vi "field_sweep_1.vi"() -> ()   [LabVIEW 2016]
uses:
  Controls/State.ctl
  Controls/Data.ctl
  <vilib>/Utility/error.llb/DialogType.ctl
  <vilib>/DAQmx/write.llb/DAQmx Write (Analog DBL 1Chan 1Samp).vi
  <vilib>/DAQmx/create/channels.llb/DAQmx Create Channel (AO-Voltage-Basic).vi
  <vilib>/DAQmx/miscellaneous.llb/DAQmx Fill In Error Info.vi
  <instrlib>/niVNA/niVNA.llb/niVNA Fetch Sweep Measurement (DBL).vi
panel:
  in  "Hysteresis":bool caption="Hysteresis On/Off"
  out "DAQ channel Out":tag="DAQ_6363/ao0"
  in  "Averaging Points":i32=10 min=1 max=3201 step=1
  in  "DAQ channel In":tag="DAQ_6363/ao0"
  in  "Exit Button":bool
  in  "IF Bandwidth":dbl(ring)=1000.0 items=["10 Hz"=10.0, "30 Hz"=30.0, "100 Hz"=100.0, "300 Hz"=300.0, "1 KHz"=1000.0, "3 KHz"=3000.0, "10 KHz"=10000.0, "30 KHz"=30000.0]
  in  "Speed (Oe/sec)":dbl=5.0
  in  "Frequency (Hz)":dbl=3000000000.0 min=10000000.0 max=6000000000.0
  in  "Save Button":bool
  out "Status":string="Shutting down...Sweeping field to zero..."
  out "Cursor":cluster{"x":dbl, "y":dbl} {"x" format="%.2f"; "y" format="%.5f"}
  out "VNA Name Out":refnum<k15>="VNA_5630"
  out "Error Out":errorcluster
  in  "Error In (no error)":errorcluster
  in  "Format":i32(ring)=1 items=["Log Magnitude (dB)"=0, "Lin Magnitude"=1, "Phase (deg)"=2, "VSWR"=3, "Group Delay"=6]
  out "SpectrumGraph":cluster{"Old Field":dbl[], "Old Signal":dbl[]}[](graph)
  in  "S-parameter":i32(ring)=1 caption="Measurement" items=["S11", "S21"]
  in  "Start Button":bool
  in  "Stop Button":bool
  in  "Output Power (dBm)":dbl=1.0 min=-25.0 max=5.0 step=0.5
  in  "Number of Points":i32=1000 min=1 max=3201 step=1
  in  "Stop H Field (Oe)":dbl=1500.0 min=-6000.0 max=6000.0 format="%#_6f"
  in  "Start H Field (Oe)":dbl=1000.0 min=-6000.0 max=6000.0 format="%#_6f"
  in  "VNA Name In":refnum<k15>="VNA_5630"
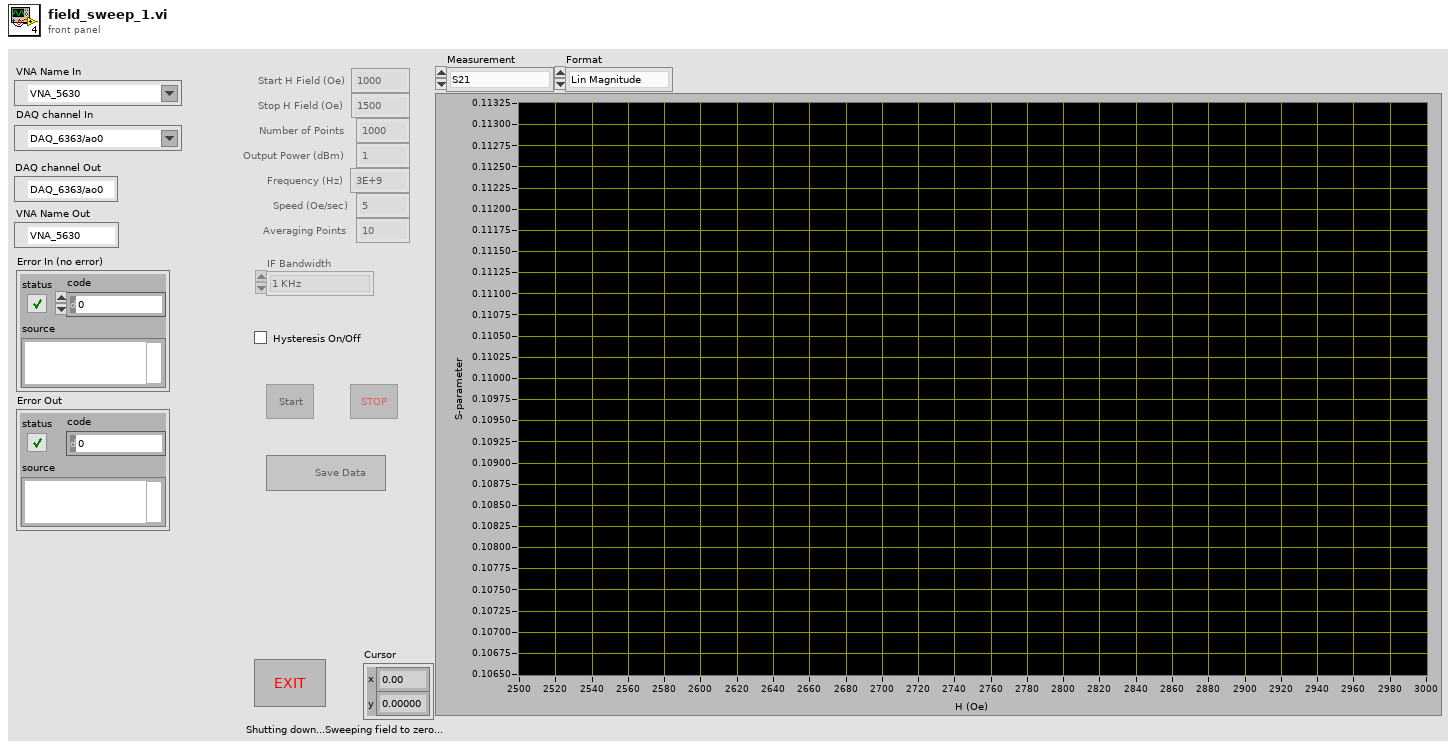
[diagram p1: front panel]
types:
  T1 = typedef "Data.ctl" = cluster{"Field":dbl[], "Signal":dbl[], "Old Field":dbl[], "Old Signal":dbl[]}
  T2 = typedef "State.ctl" = enum16{"Init", "Idle", "Sweeping up", "Sweeping down", "Running", "Shutdown"}
  T3 = typedef "DialogType.ctl" = u16
  T4 = typedef "LVPoint32TypeDef.ctl" = cluster{"Horizontal":i32, "Vertical":i32}
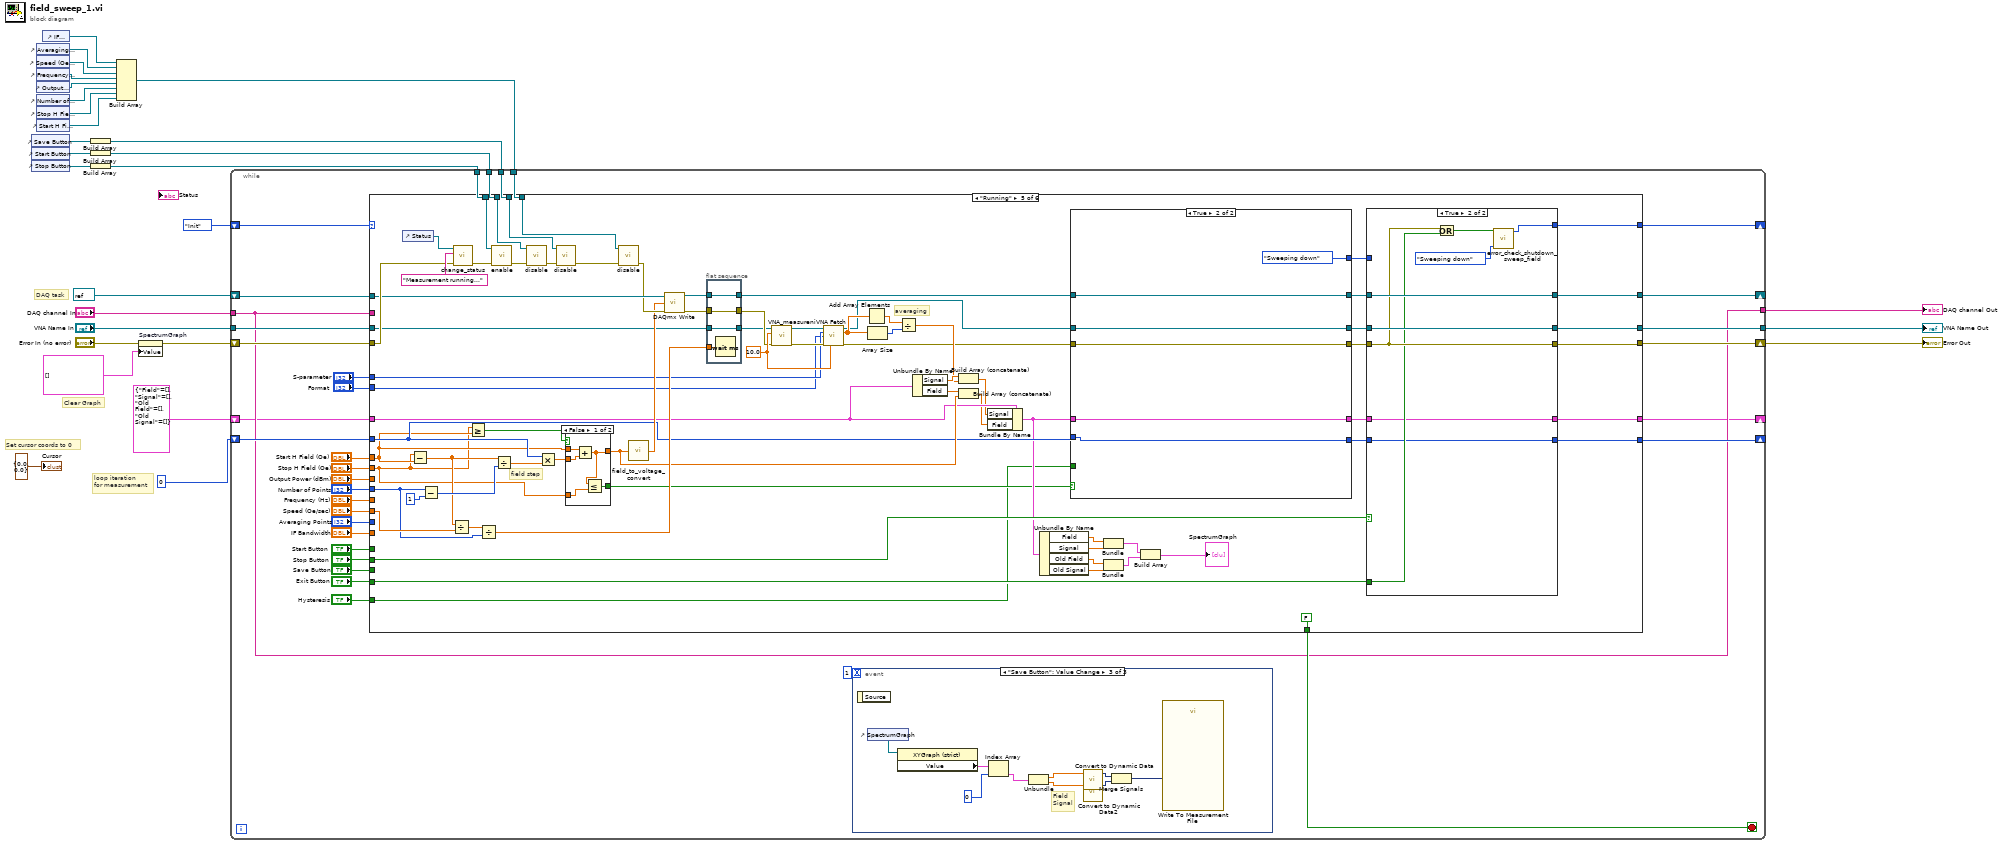
[diagram p0: block diagram]
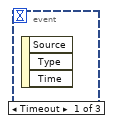
[diagram p2: hidden frame]
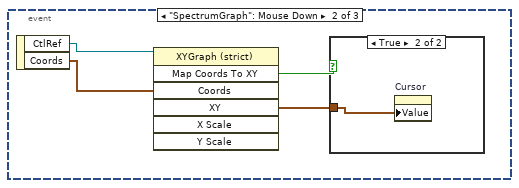
[diagram p3: hidden frame]
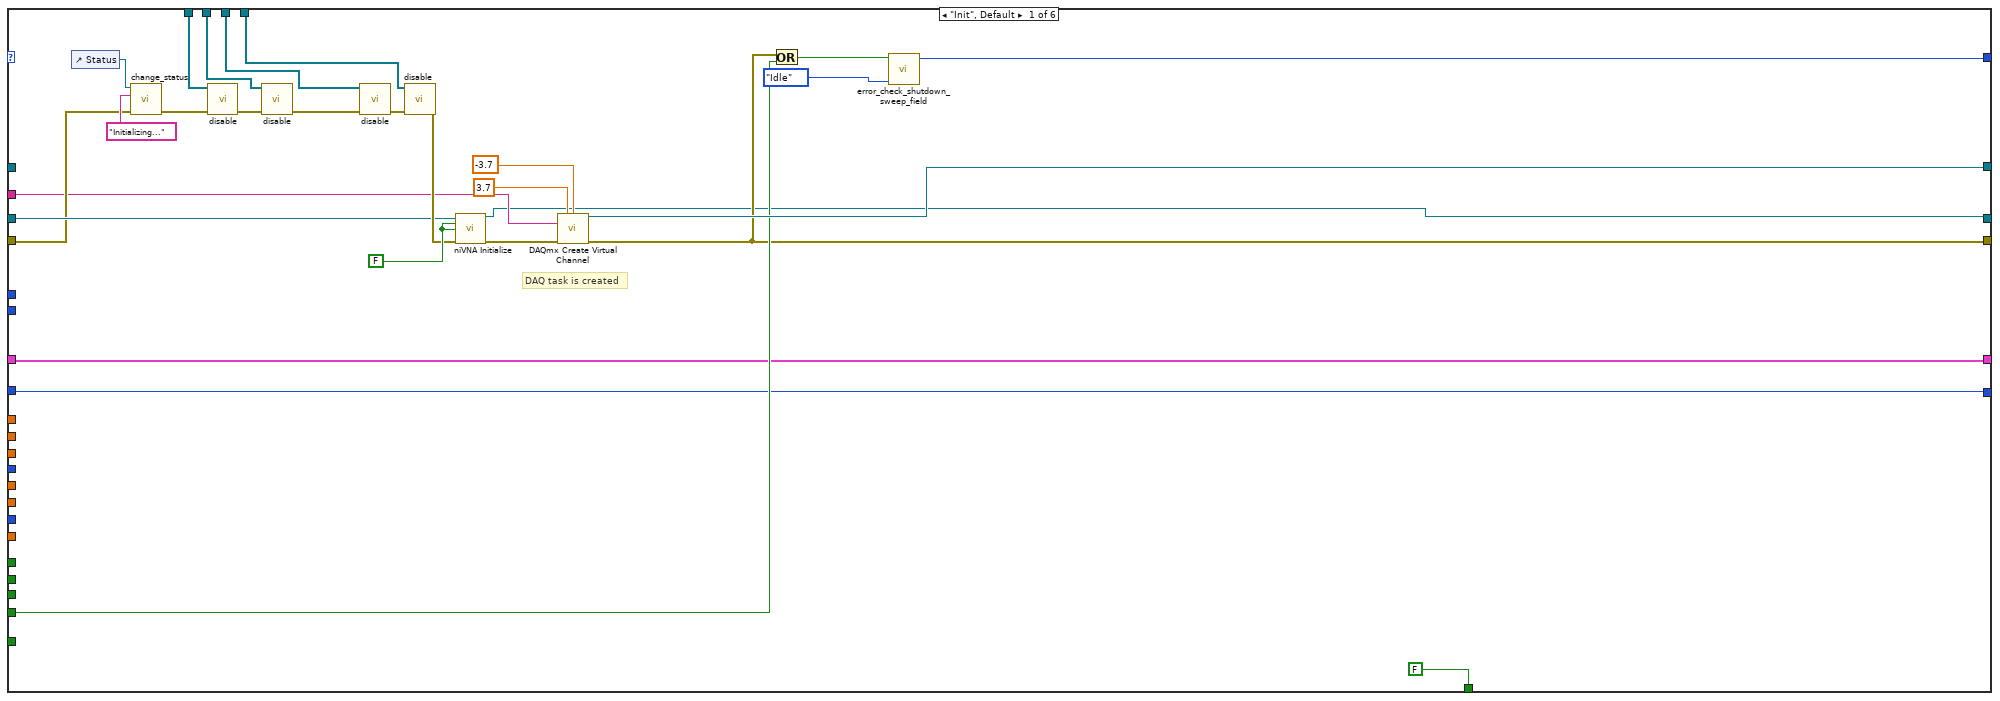
[diagram p5: hidden frame]
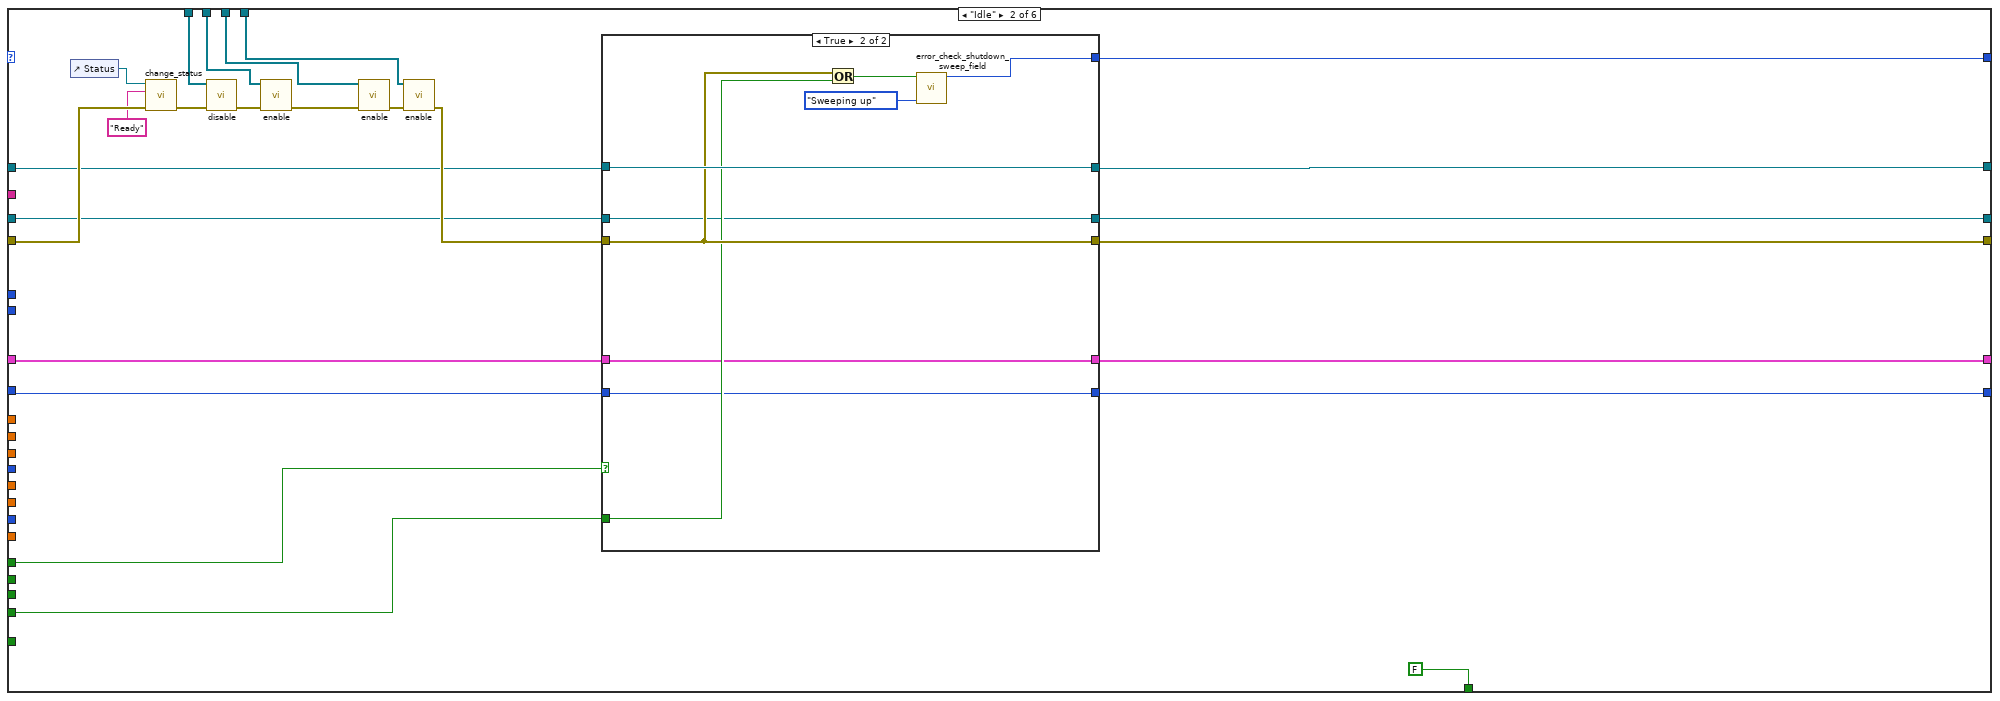
[diagram p6: hidden frame]
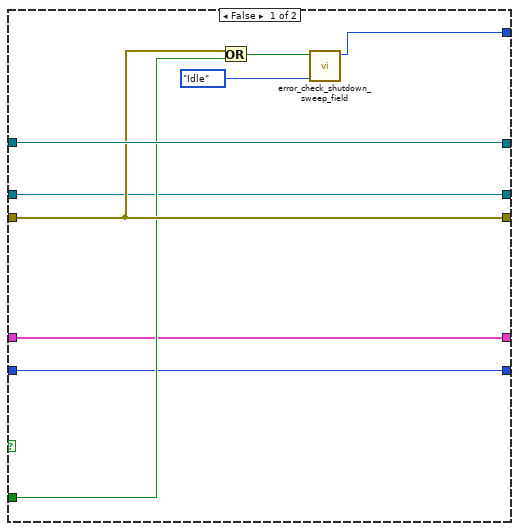
[diagram p7: hidden frame]
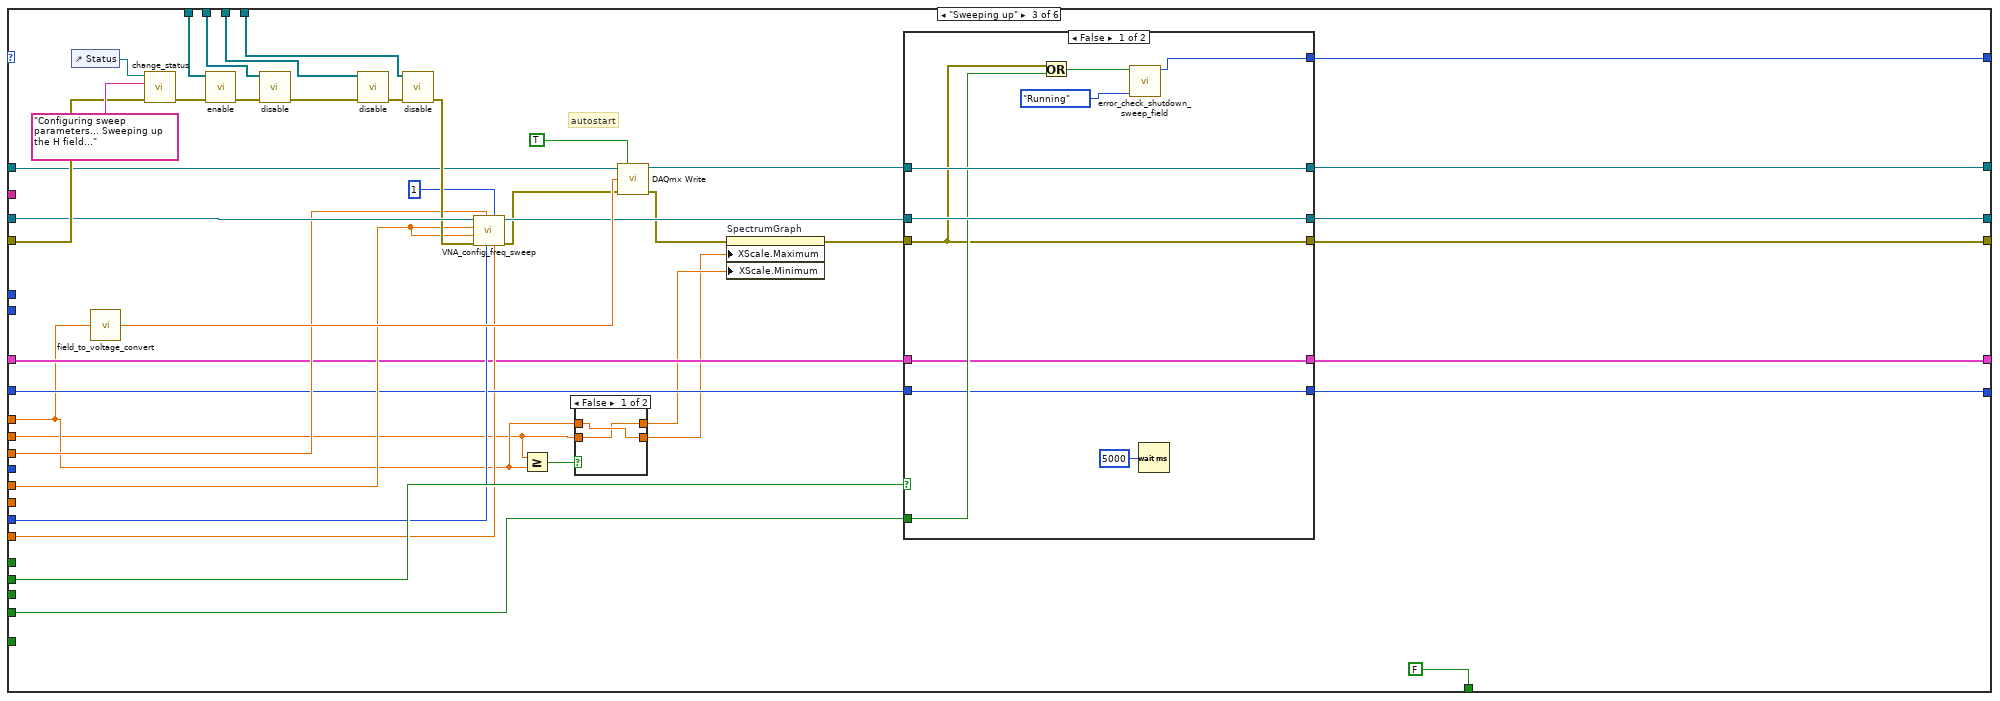
[diagram p8: hidden frame]
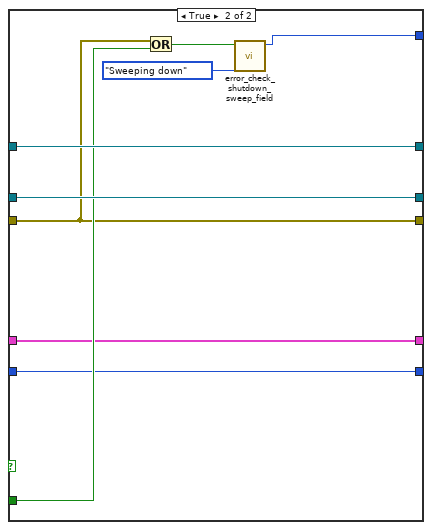
[diagram p10: hidden frame]
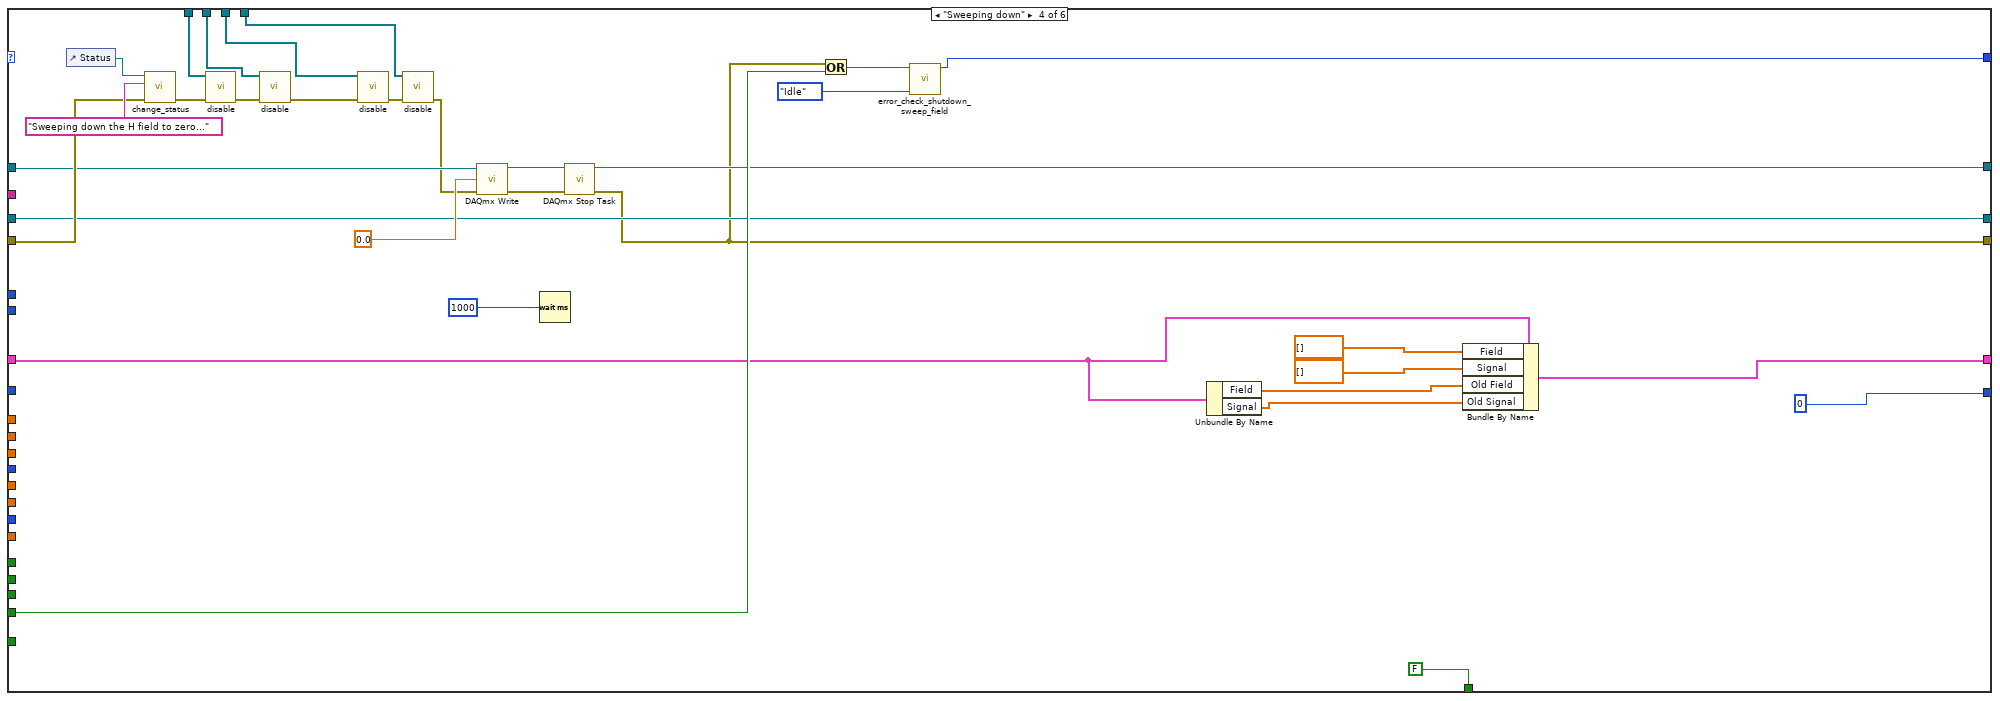
[diagram p11: hidden frame]
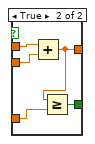
[diagram p12: hidden frame]
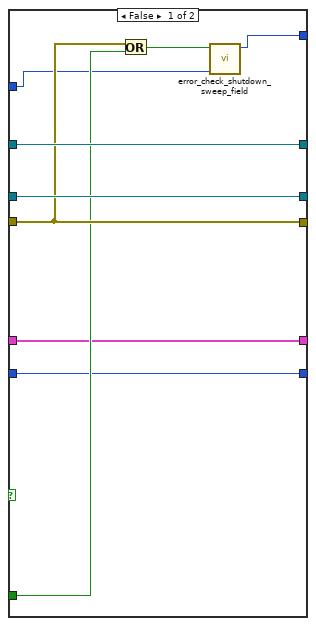
[diagram p13: hidden frame]
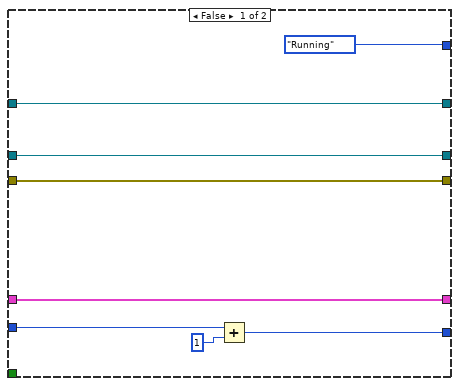
[diagram p14: hidden frame]
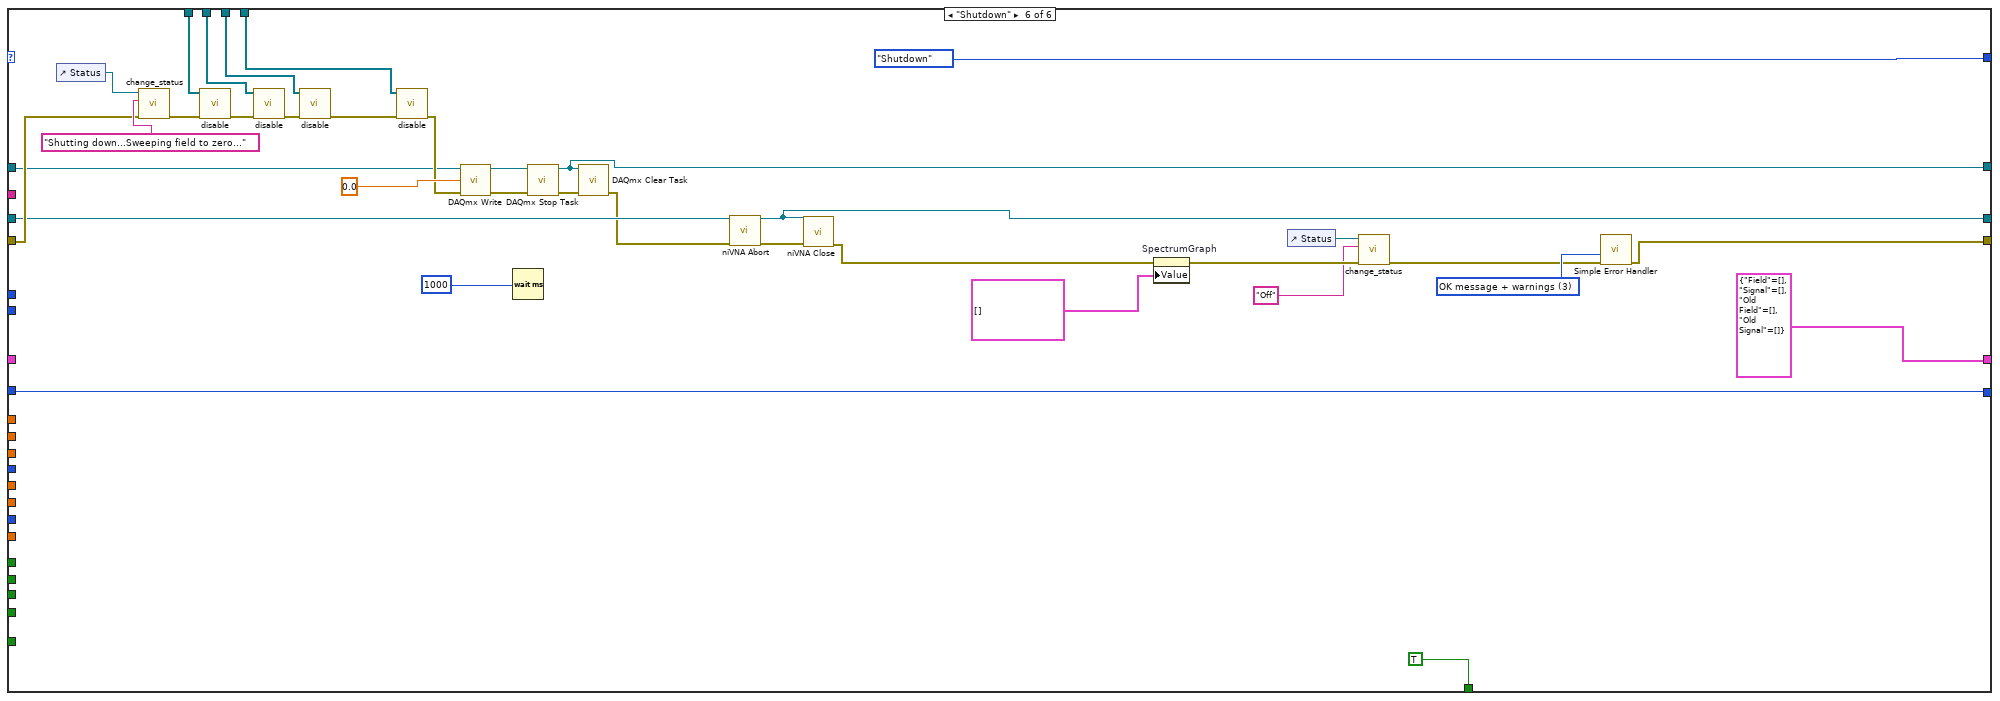
[diagram p15: hidden frame]
diagram:
  # "loop iteration\nfor measurement"
  # "DAQ task"
  # "Set cursor coords to 0"
  # "Clear Graph"
  n1 = control-ref of="Save Button"() -> (w11:refnum<vi>)
  n2 = control-ref of="Start Button"() -> (w19:refnum<vi>)
  n3 = control-ref of="Stop Button"() -> (w18:refnum<vi>)
  n4 = control-ref of="Averaging Points"() -> (w8:refnum<vi>)
  n5 = control-ref of="Speed (Oe/sec)"() -> (w25:refnum<vi>)
  n6 = control-ref of="Frequency (Hz)"() -> (w24:refnum<vi>)
  n7 = control-ref of="Output Power (dBm)"() -> (w23:refnum<vi>)
  n8 = control-ref of="Number of Points"() -> (w22:refnum<vi>)
  n9 = control-ref of="Stop H Field (Oe)"() -> (w21:refnum<vi>)
  n10 = control-ref of="Start H Field (Oe)"() -> (w20:refnum<vi>)
  n11 = control-ref of="IF Bandwidth"() -> (w26:refnum<vi>)
  n12 = Build Array(w11) -> (w10:refnum<vi>[])
  n13 = Build Array(w19) -> (w16:refnum<vi>[])
  n14 = Build Array(w18) -> (w15:refnum<vi>[])
  n15 = Build Array(w26, w8, w25, w24, w23, w22, w21, w20) -> (w17:refnum<vi>[])
  n16 = property on="SpectrumGraph" class="XYGraph (strict)"(error in="Error In (no error)", "Value"=cluster{"Old Field":dbl[], "Old Signal":dbl[]}[] [] ("SpectrumGraph")) -> (error out=w4:errorcluster)  [unwired: 1 in, 1 out]
  n17 = while {
    shift-right: [w57] -> _
    shift-left: State."Init" -> [w62]
    shift-right: [w37] -> _
    shift-left: 0 -> [w39]
    tunnel: w17 -> [w61]
    tunnel: w16 -> [w60]
    tunnel: w15 -> [w59]
    tunnel: "VNA Name In" -> [w58]
    tunnel: "DAQ channel In" -> [w36]
    shift-right: [w56] -> w1
    shift-left: w4 -> [w55]
    shift-right: [w54] -> _
    shift-left: refnum<k21> refnum ("task in") -> [w53]
    tunnel: w10 -> [w52]
    tunnel: [w40] -> w7
    shift-right: [w32] -> _
    shift-left: T1 {"Field"=[], "Signal"=[], "Old Field"=[], "Old Signal"=[]} ("Cluster") -> [w33]
    tunnel: [w36] -> w6
    stop <- w47 stop-if-true
    n18 = case shown="\"Running\"" w62 {
      tunnel: w61 -> [w88 w126 w181 w235 w311 w391]
      tunnel: w60 -> [w102 w128 w183 w233 w313 w393]
      tunnel: w59 -> [w104 w129 w184 w232 w315 w394]
      tunnel: w58 -> [w96 w115 w170 w228 w282 w375]
      tunnel: w55 -> [w95 w121 w179 w239 w309 w389]
      tunnel: [w84 w112 w172 w229 w266 State."Shutdown"] -> w57
      tunnel: w36 -> [w91 _ _ _ _ _]
      tunnel: [w83 w116 w177 w221 w272 w384] -> w56
      tunnel: [w90 w113 w175 w223 w276 w385] -> w54
      tunnel: w53 -> [_ w114 w155 w237 w308 w378]
      tunnel: w52 -> [w89 w127 w182 w234 w312 w392]
      tunnel: "Start Button" -> [_ w118 _ _ _ _]
      tunnel: "Stop Button" -> [_ _ w178 _ w271 _]
      tunnel: "Save Button" -> [_ _ _ _ _ _]
      tunnel: "Exit Button" -> [w85 w111 w171 w230 w270 _]
      tunnel: [FALSE FALSE FALSE FALSE FALSE TRUE] -> w47
      tunnel: "Start H Field (Oe)" -> [_ _ w151 _ w251 _]
      tunnel: "Stop H Field (Oe)" -> [_ _ w150 _ w249 _]
      tunnel: "Output Power (dBm)" -> [_ _ w166 _ _ _]
      tunnel: "Number of Points" -> [_ _ _ _ w294 _]
      tunnel: "Frequency (Hz)" -> [_ _ w167 _ _ _]
      tunnel: "Speed (Oe/sec)" -> [_ _ _ _ w296 _]
      tunnel: [w81 w110 w176 w228 w274 w386] -> w40
      tunnel: w39 -> [w80 w108 w164 _ w278 w373]
      tunnel: "Averaging Points" -> [_ _ w165 _ _ _]
      tunnel: [w80 w109 w163 0 w268 w373] -> w37
      tunnel: "IF Bandwidth" -> [_ _ w159 _ _ _]
      tunnel: [w78 w105 w156 w219 w260 T1 {"Field"=[], "Signal"=[], "Old Field"=[], "Old Signal"=[]} ("Cluster")] -> w32
      tunnel: w33 -> [w78 w106 w157 w216 w264 _]
      tunnel: "Hysteresis" -> [_ _ _ _ w247 _]
      tunnel: "S-parameter" -> [_ _ _ _ w246 _]
      tunnel: "Format" -> [_ _ _ _ w245 _]
      frame "Init", Default {
        w98 = FALSE ("id query")
        # "DAQ task is created"
        n19 = control-ref of="Status"() -> (w100:refnum<vi>)
        n20 = call "change_status.vi"("error in (no error)"=w95, "String"="Initializing...", "String in"=w100) -> ("error out"=w101:errorcluster)  [unwired: 8 in]
        n21 = call "disable.vi"("error in (no error)"=w101, "Array"=w104) -> ("error out"=w103:errorcluster)  [unwired: 9 in]
        n22 = call "disable.vi"("error in (no error)"=w103, "Array"=w102) -> ("error out"=w87:errorcluster)  [unwired: 9 in]
        n23 = call "disable.vi"("error in (no error)"=w87, "Array"=w89) -> ("error out"=w86:errorcluster)  [unwired: 9 in]
        n24 = call "disable.vi"("error in (no error)"=w86, "Array"=w88) -> ("error out"=w97:errorcluster)  [unwired: 9 in]
        n25 = call <instrlib>:"niVNA Initialize.vi"("resource name"=w96, "id query"=w98, "reset"=w98, "error in"=w97) -> ("instrument handle"=w81:refnum<k15>, "error out"=w94:errorcluster)  [unwired: 10 in]
        n26 = call-poly <vilib>:"DAQmx Create Virtual Channel.vi"("maximum value"=3.7, "minimum value"=-3.7, "physical channels"=w91, "error in"=w94) -> ("task out"=w90:refnum<k21>, "error out"=w83:errorcluster)  [unwired: 10 in]
        n27 = Or(x=w83, y=w85) -> (x .or. y?=w82:bool)
        n28 = call "error_check_shutdown_sweep_field.vi"("State In"=State."Idle", "Boolean"=w82) -> ("State Out"=w84:T2)  [unwired: 9 in]
      }
      frame "Idle" {
        n29 = control-ref of="Status"() -> (w120:refnum<vi>)
        n30 = call "change_status.vi"("error in (no error)"=w121, "String"="Ready", "String in"=w120) -> ("error out"=w122:errorcluster)  [unwired: 8 in]
        n31 = call "disable.vi"("error in (no error)"=w122, "Array"=w129) -> ("error out"=w125:errorcluster)  [unwired: 9 in]
        n32 = call "enable.vi"("error in (no error)"=w125, "Array"=w128) -> ("error out"=w124:errorcluster)  [unwired: 9 in]
        n33 = call "enable.vi"("error in (no error)"=w124, "Array"=w127) -> ("error out"=w123:errorcluster)  [unwired: 9 in]
        n34 = call "enable.vi"("error in (no error)"=w123, "Array"=w126) -> ("error out"=w117:errorcluster)  [unwired: 9 in]
        n35 = case shown="True" w118 {
          tunnel: w117 -> [w135 w145]
          tunnel: [w135 w145] -> w116
          tunnel: w115 -> [w133 w142]
          tunnel: w114 -> [w138 w147]
          tunnel: [w138 w147] -> w113
          tunnel: [w136 w143] -> w112
          tunnel: w111 -> [w134 w144]
          tunnel: [w133 w142] -> w110
          tunnel: [w132 w141] -> w109
          tunnel: w108 -> [w132 w141]
          tunnel: w106 -> [w131 w140]
          tunnel: [w131 w140] -> w105
          frame False {
            n36 = Or(x=w135, y=w134) -> (x .or. y?=w137:bool)
            n37 = call "error_check_shutdown_sweep_field.vi"("State In"=State."Idle", "Boolean"=w137) -> ("State Out"=w136:T2)  [unwired: 9 in]
          }
          frame True {
            n38 = Or(x=w145, y=w144) -> (x .or. y?=w146:bool)
            n39 = call "error_check_shutdown_sweep_field.vi"("State In"=State."Sweeping up", "Boolean"=w146) -> ("State Out"=w143:T2)  [unwired: 9 in]
          }
        }
      }
      frame "Sweeping up" {
        # "autostart"
        n40 = control-ref of="Status"() -> (w180:refnum<vi>)
        n41 = call "field_to_voltage_convert.vi"("Start H Field (Oe)"=w151) -> ("Numeric"=w173:dbl)
        n42 = call "change_status.vi"("error in (no error)"=w179, "String"="Configuring sweep parameters... Sweeping up the H field...", "String in"=w180) -> ("error out"=w188:errorcluster)  [unwired: 8 in]
        n43 = call "enable.vi"("error in (no error)"=w188, "Array"=w184) -> ("error out"=w187:errorcluster)  [unwired: 9 in]
        n44 = call "disable.vi"("error in (no error)"=w187, "Array"=w183) -> ("error out"=w186:errorcluster)  [unwired: 9 in]
        n45 = call "disable.vi"("error in (no error)"=w186, "Array"=w182) -> ("error out"=w185:errorcluster)  [unwired: 9 in]
        n46 = call "disable.vi"("error in (no error)"=w185, "Array"=w181) -> ("error out"=w169:errorcluster)  [unwired: 9 in]
        n47 = call "VNA_config_freq_sweep.vi"("IF Bandwidth"=w159, "Averaging"=1, "Number of Points"=w165, "Output Power"=w166, "error in (no error)"=w169, "Stop Frequency"=w167, "Start Frequency"=w167, "Resource Name In"=w170) -> ("error out"=w154:errorcluster, "Resource Name Out"=w168:refnum<k15>)  [unwired: 2 in]
        n48 = Greater Or Equal?(x=w150, y=w151) -> (x >= y?=w152:bool)
        n49 = case shown="False" w152 {
          tunnel: w151 -> [w191 w193]
          tunnel: w150 -> [w190 w192]
          tunnel: [w190 w193] -> w149
          tunnel: [w191 w192] -> w148
          frame False {
          }
          frame True {
          }
        }
        n50 = call-poly <vilib>:"DAQmx Write.vi"("task/channels in"=w155, "auto start"=TRUE, "data"=w173, "error in"=w154) -> ("task out"=w174:refnum<k21>, "error out"=w161:errorcluster)  [unwired: 9 in, 1 out]
        n51 = property on="SpectrumGraph" class="XYGraph (strict)"(error in=w161, "XScale.Maximum"=w148, "XScale.Minimum"=w149) -> (error out=w160:errorcluster)  [unwired: 1 in, 1 out]
        n52 = case shown="False" w178 {
          tunnel: w160 -> [w198 w207]
          tunnel: w174 -> [w203 w211]
          tunnel: w168 -> [w202 w212]
          tunnel: [w198 w207] -> w177
          tunnel: [w202 w212] -> w176
          tunnel: [w203 w211] -> w175
          tunnel: [w200 w209] -> w172
          tunnel: w171 -> [w199 w208]
          tunnel: w164 -> [w196 w206]
          tunnel: [w196 w206] -> w163
          tunnel: w157 -> [w195 w205]
          tunnel: [w195 w205] -> w156
          frame False {
            n53 = Or(x=w198, y=w199) -> (x .or. y?=w201:bool)
            n54 = call "error_check_shutdown_sweep_field.vi"("State In"=State."Running", "Boolean"=w201) -> ("State Out"=w200:T2)  [unwired: 9 in]
            n55 = Wait (ms)(milliseconds to wait=u32 5000) -> ()  [unwired: 1 out]
          }
          frame True {
            n56 = Or(x=w207, y=w208) -> (x .or. y?=w210:bool)
            n57 = call "error_check_shutdown_sweep_field.vi"("State In"=State."Sweeping down", "Boolean"=w210) -> ("State Out"=w209:T2)  [unwired: 9 in]
          }
        }
      }
      frame "Sweeping down" {
        n58 = control-ref of="Status"() -> (w227:refnum<vi>)
        n59 = call "change_status.vi"("error in (no error)"=w239, "String"="Sweeping down the H field to zero...", "String in"=w227) -> ("error out"=w243:errorcluster)  [unwired: 8 in]
        n60 = call "disable.vi"("error in (no error)"=w243, "Array"=w232) -> ("error out"=w242:errorcluster)  [unwired: 9 in]
        n61 = call "disable.vi"("error in (no error)"=w242, "Array"=w233) -> ("error out"=w241:errorcluster)  [unwired: 9 in]
        n62 = call "disable.vi"("error in (no error)"=w241, "Array"=w234) -> ("error out"=w240:errorcluster)  [unwired: 9 in]
        n63 = call "disable.vi"("error in (no error)"=w240, "Array"=w235) -> ("error out"=w236:errorcluster)  [unwired: 9 in]
        n64 = call-poly <vilib>:"DAQmx Write.vi"("task/channels in"=w237, "data"=0.0, "error in"=w236) -> ("task out"=w224:refnum<k21>, "error out"=w222:errorcluster)  [unwired: 10 in, 1 out]
        n65 = Wait (ms)(milliseconds to wait=u32 1000) -> ()  [unwired: 1 out]
        n66 = call <vilib>:"DAQmx Stop Task.vi"("task/channels in"=w224, "error in"=w222) -> ("task out"=w223:refnum<k21>, "error out"=w221:errorcluster)  [unwired: 12 in]
        n67 = Or(x=w221, y=w230) -> (x .or. y?=w231:bool)
        n68 = call "error_check_shutdown_sweep_field.vi"("State In"=State."Idle", "Boolean"=w231) -> ("State Out"=w229:T2)  [unwired: 9 in]
        n69 = Unbundle By Name(w216) -> ("Field"=w215:dbl[], "Signal"=w214:dbl[])
        n70 = Bundle By Name(cluster=w216, "Field"=dbl[] [], "Signal"=dbl[] [], "Old Field"=w215, "Old Signal"=w214) -> (w219:T1)
      }
      frame "Running" {
        w302 = 10.0 ("timeout")
        # "averaging"
        # "field step"
        n71 = control-ref of="Status"() -> (w310:refnum<vi>)
        n72 = Subtract(x=w249, y=w251) -> (x-y=w288:dbl)
        n73 = Subtract(x=w294, y=1) -> (x-y=w305:i32)
        n74 = Divide(x=w288, y=w296) -> (x/y=w295:dbl)
        n75 = call "change_status.vi"("error in (no error)"=w309, "String"="Measurement running...", "String in"=w310) -> ("error out"=w316:errorcluster)  [unwired: 8 in]
        n76 = Greater Or Equal?(x=w249, y=w251) -> (x >= y?=w250:bool)
        n77 = Divide(x=w295, y=w294) -> (x/y=w293:dbl)
        n78 = call "enable.vi"("error in (no error)"=w316, "Array"=w315) -> ("error out"=w319:errorcluster)  [unwired: 9 in]
        n79 = Divide(x=w288, y=w305) -> (x/y=w304:dbl)
        n80 = call "disable.vi"("error in (no error)"=w319, "Array"=w313) -> ("error out"=w318:errorcluster)  [unwired: 9 in]
        n81 = Multiply(x=w278, y=w304) -> (x*y=w303:dbl)
        n82 = call "disable.vi"("error in (no error)"=w318, "Array"=w312) -> ("error out"=w317:errorcluster)  [unwired: 9 in]
        n83 = case shown="False" w250 {
          tunnel: w303 -> [w323 w329]
          tunnel: w251 -> [w324 w328]
          tunnel: [w321 w326] -> w284
          tunnel: w249 -> [w322 w325]
          tunnel: [w320 w327] -> w248
          frame False {
            n84 = Add(x=w324, y=w323) -> (x+y=w321:dbl)
            n85 = Less Or Equal?(x=w321, y=w322) -> (x <= y?=w320:bool)
          }
          frame True {
            n86 = Add(x=w328, y=w329) -> (x+y=w326:dbl)
            n87 = Greater Or Equal?(x=w326, y=w325) -> (x >= y?=w327:bool)
          }
        }
        n88 = call "disable.vi"("error in (no error)"=w317, "Array"=w311) -> ("error out"=w307:errorcluster)  [unwired: 9 in]
        n89 = call "field_to_voltage_convert.vi"("Start H Field (Oe)"=w284) -> ("Numeric"=w289:dbl)
        n90 = call-poly <vilib>:"DAQmx Write.vi"("task/channels in"=w308, "data"=w289, "error in"=w307) -> ("task out"=w292:refnum<k21>, "error out"=w291:errorcluster)  [unwired: 10 in, 1 out]
        n91 = flat-sequence {
          tunnel: w293 -> [w365]
          tunnel: w292 -> [w364]
          tunnel: [w364] -> w283
          tunnel: w291 -> [w363]
          tunnel: [w363] -> w290
          tunnel: w282 -> [w362]
          tunnel: [w362] -> w281
          frame #0 {
            n92 = Wait (ms)(milliseconds to wait=w365) -> ()  [unwired: 1 out]
          }
        }
        n93 = call "VNA_measure.vi"("error in (no error)"=w290, "timeout"=w302, "Resource Name In"=w281) -> ("error out"=w301:errorcluster, "Resource Name Out"=w300:refnum<k15>)  [unwired: 7 in]
        n94 = call-poly <instrlib>:"niVNA Fetch.vi"("instrument handle"=w300, "measurement"=w246, "format"=w245, "error in"=w301, "timeout"=w302) -> ("instrument handle out"=w280:refnum<k15>, "data"=w299:dbl[], "error out"=w279:errorcluster)  [unwired: 7 in, 1 out]
        n95 = Add Array Elements(numeric array=w299) -> (sum=w298:dbl)
        n96 = Array Size(array=w299) -> (size(s)=w297:i32)
        n97 = Divide(x=w298, y=w297) -> (x/y=w286:dbl)
        n98 = Unbundle By Name(w264) -> ("Signal"=w287:dbl[], "Field"=w285:dbl[])
        n99 = Build Array (concatenate)(w287, w286) -> (w263:dbl[])
        n100 = Build Array (concatenate)(w285, w284) -> (w262:dbl[])
        n101 = Bundle By Name(cluster=w264, "Signal"=w263, "Field"=w262) -> (w259:T1)
        n102 = Unbundle By Name(w259) -> ("Field"=w258:dbl[], "Signal"=w257:dbl[], "Old Field"=w256:dbl[], "Old Signal"=w255:dbl[])
        n103 = case shown="True" w248 {
          tunnel: [State."Running" State."Sweeping down"] -> w267
          tunnel: w283 -> [w354 w359]
          tunnel: [w354 w359] -> w277
          tunnel: w280 -> [w353 w360]
          tunnel: [w353 w360] -> w275
          tunnel: w279 -> [w352 w358]
          tunnel: [w352 w358] -> w273
          tunnel: w278 -> [w351 w357]
          tunnel: [w349 w357] -> w269
          tunnel: w259 -> [w348 w356]
          tunnel: [w348 w356] -> w261
          tunnel: w247 -> [_ _]
          frame False {
            n104 = Add(x=w351, y=1) -> (x+y=w349:i32)
          }
          frame True {
          }
        }
        n105 = Bundle("Field"=w258, "Signal"=w257) -> (w254:cluster{"Field":dbl[], "Signal":dbl[]})  [unwired: 1 in]
        n106 = Bundle("Old Field"=w256, "Old Signal"=w255) -> (w253:cluster{"Old Field":dbl[], "Old Signal":dbl[]})  [unwired: 1 in]
        n107 = Build Array(w254, w253) -> (→"SpectrumGraph":cluster{"Old Field":dbl[], "Old Signal":dbl[]}[])
        n108 = case shown="True" w271 {
          tunnel: [w337 w346] -> w266
          tunnel: w277 -> [w336 w345]
          tunnel: [w336 w345] -> w276
          tunnel: w275 -> [w335 w344]
          tunnel: [w335 w344] -> w274
          tunnel: w273 -> [w334 w343]
          tunnel: [w334 w343] -> w272
          tunnel: w270 -> [w333 w342]
          tunnel: w269 -> [w332 w341]
          tunnel: [w332 w341] -> w268
          tunnel: w267 -> [w330 _]
          tunnel: [w331 w340] -> w260
          tunnel: w261 -> [w331 w340]
          frame False {
            n109 = Or(x=w334, y=w333) -> (x .or. y?=w338:bool)
            n110 = call "error_check_shutdown_sweep_field.vi"("State In"=w330, "Boolean"=w338) -> ("State Out"=w337:T2)  [unwired: 9 in]
          }
          frame True {
            n111 = Or(x=w343, y=w342) -> (x .or. y?=w347:bool)
            n112 = call "error_check_shutdown_sweep_field.vi"("State In"=State."Sweeping down", "Boolean"=w347) -> ("State Out"=w346:T2)  [unwired: 9 in]
          }
        }
      }
      frame "Shutdown" {
        w383 = T3 3 items=["no dialog", "OK message", "continue or stop message", "OK message + warnings", "continue/stop + warnings"] ("type of dialog (OK msg:1)")
        n113 = control-ref of="Status"() -> (w390:refnum<vi>)
        n114 = call "change_status.vi"("error in (no error)"=w389, "String"="Shutting down...Sweeping field to zero...", "String in"=w390) -> ("error out"=w396:errorcluster)  [unwired: 8 in]
        n115 = call "disable.vi"("error in (no error)"=w396, "Array"=w394) -> ("error out"=w399:errorcluster)  [unwired: 9 in]
        n116 = call "disable.vi"("error in (no error)"=w399, "Array"=w393) -> ("error out"=w398:errorcluster)  [unwired: 9 in]
        n117 = call "disable.vi"("error in (no error)"=w398, "Array"=w392) -> ("error out"=w397:errorcluster)  [unwired: 9 in]
        n118 = call "disable.vi"("error in (no error)"=w397, "Array"=w391) -> ("error out"=w379:errorcluster)  [unwired: 9 in]
        n119 = call-poly <vilib>:"DAQmx Write.vi"("task/channels in"=w378, "data"=0.0, "error in"=w379) -> ("task out"=w376:refnum<k21>, "error out"=w377:errorcluster)  [unwired: 10 in, 1 out]
        n120 = Wait (ms)(milliseconds to wait=u32 1000) -> ()  [unwired: 1 out]
        n121 = call <vilib>:"DAQmx Stop Task.vi"("task/channels in"=w376, "error in"=w377) -> ("task out"=w385:refnum<k21>, "error out"=w387:errorcluster)  [unwired: 12 in]
        n122 = call <vilib>:"DAQmx Clear Task.vi"("task in"=w385, "error in"=w387) -> ("error out"=w374:errorcluster)  [unwired: 13 in]
        n123 = call <instrlib>:"niVNA Abort.vi"("instrument handle"=w375, "error in"=w374) -> ("instrument handle out"=w386:refnum<k15>, "error out"=w388:errorcluster)  [unwired: 12 in]
        n124 = call <instrlib>:"niVNA Close.vi"("instrument handle"=w386, "error in"=w388) -> ("error out"=w371:errorcluster)  [unwired: 13 in]
        n125 = property on="SpectrumGraph" class="XYGraph (strict)"(error in=w371, "Value"=cluster{"Old Field":dbl[], "Old Signal":dbl[]}[] [] ("SpectrumGraph")) -> (error out=w369:errorcluster)  [unwired: 1 in, 1 out]
        n126 = control-ref of="Status"() -> (w366:refnum<vi>)
        n127 = call "change_status.vi"("error in (no error)"=w369, "String"="Off", "String in"=w366) -> ("error out"=w368:errorcluster)  [unwired: 8 in]
        n128 = call <vilib>:"Simple Error Handler.vi"("type of dialog (OK msg:1)"=w383, "error in (no error)"=w368) -> ("error out"=w384:errorcluster)  [unwired: 3 in, 4 out]
      }
    }
    n129 = event shown="[2] \"Save Button\": Value Change" {
      selector: _ -> [_ _ _]
      dyn-events: _ -> [_ _ _]
      timeout: 1 -> [_ _ _]
      event Timeout {
        n130 = event-data() -> ()  [unwired: 1 in, 3 out]
      }
      event "SpectrumGraph": Mouse Down {
        n131 = event-data() -> ("CtlRef"=w64:refnum<vi>, "Coords"=w63:T4)  [unwired: 1 in]
        n132 = invoke on="Invoke Node" class="XYGraph (strict)" method="Map Coords To XY"(reference=w64, "Coords"=w63) -> ("Map Coords To XY"=w65:bool, "XY"=w66:cluster{"X":dbl, "Y":dbl})  [unwired: 5 in, 5 out]
        n133 = case shown="True" w65 {
          tunnel: w66 -> [_ w67]
          frame False {
          }
          frame True {
            n134 = property on="Cursor" class="Clust (strict)"("Value"=w67) -> ()  [unwired: 2 in, 2 out]
          }
        }
      }
      event "Save Button": Value Change {
        # "Field\nSignal"
        n135 = event-data() -> ()  [unwired: 1 in, 1 out]
        n136 = control-ref of="SpectrumGraph"() -> (w76:refnum<vi>)
        n137 = property class="XYGraph (strict)"(reference=w76) -> ("Value"=w74:cluster{"Old Field":dbl[], "Old Signal":dbl[]}[])  [unwired: 1 in, 2 out]
        n138 = Index Array(array=w74, index=0) -> (element=w73:cluster{"Old Field":dbl[], "Old Signal":dbl[]})
        n139 = Unbundle(w73) -> ("Old Field"=w72:dbl[], "Old Signal"=w69:dbl[])
        n140 = call "Convert to Dynamic Data"("Array"=w72) -> ("Dynamic Data Type"=w71:dynamicdata)  [unwired: 3 in]
        n141 = call "Convert to Dynamic Data2"("Array"=w69) -> ("Dynamic Data Type"=w68:dynamicdata)  [unwired: 3 in]
        n142 = Merge Signals(w71, w68) -> (w70:dynamicdata)
        n143 = call "Write To Measurement File"("Signals"=w70) -> ()  [unwired: 16 in, 3 out]
      }
    }
  }
  "Error Out" <- w1
  "VNA Name Out" <- w7
  "DAQ channel Out" <- w6
  "Cursor" <- cluster{"x":dbl, "y":dbl} {"x"=0.0, "y"=0.0} ("Cursor")
